vi "Verarbeitung_Unten.vi"(8 "Fehler in":errorcluster, 11 "Cluster in":T2={"Initialisierung"={"Online?"=FALSE, "Grundpfad"=path "", "Kamera Oben"="", "IP-Adresse Flüssiglinse"="", "Flüssiglinse"=refnum, "Kamera Unten"="", "IP-Adresse SPS"="", "SPS-Verbindung"={"TCP Connection Ref"=refnum, "IP address"="", "timeout ms"=5000, "Connected?"=FALSE, "PLC Type"=enum."S7 1200", "Rack S7 400"=0, "Slot S7 400"=0, "PDU Size"=0, "connection semaphore"=refnum}, "IP-Adresse Lichtgitter"="", "Lichtgitter"=refnum, "Skalierungsfaktor"=0.0, "Bilder Oben"=[], "Bild Unten"=refnum, "Bild Ausschnitt Unten"=refnum}, "Einstellungen"={"Gesamtablauf gestartet"=FALSE, "i. O. Bilder speichern"=FALSE, "Bildspeicherung Offline"=FALSE, "Ausgewähltes Offline-Datum"="", "Ausgewähltes Offline-Teil"="", "Speicherpfad Bilder"=path ""}, "Artikeldaten"={"Artikelnummer"="", "Fertigungsauftrag"="", "Muster ISO"=refnum, "Belichtungszeit Referenzmarken"=0.0, "Fokus Referenzmarken"=0.0, "Belichtungszeit ISO"=0.0, "Fokus ISO"=0.0, "Belichtungszeit Unten"=0.0, "Kontaktanzahl"=0, "Aktueller Kontakt"=0, "Kontaktposition"={"x"=0.0, "y"=0.0}, "Winkel ISO"=0.0, "ISO-Muster nicht vorhanden"=FALSE}, "Werte Kamera Oben"={"Koordinatensystem"={"Punkt x-Achse"={"X"=0.0, "Y"=0.0}, "Ursprung"={"X"=0.0, "Y"=0.0}, "Punkt y-Achse"={"X"=0.0, "Y"=0.0}}, "Position Kontakt"={"x"=0.0, "y"=0.0}, "Winkel Kontakt"=0.0}, "Werte Kamera Unten"={"Prüfung Unten n. i. O."=FALSE}, "Werte Lichtgitter"={"Messwerte Referenzmarken"=[], "Mittelpunkt Referenzmarken"={"x"=0.0, "y"=0.0}, "Messwerte Kontakt"=[], "Offset"={"x"=0.0, "y"=0.0}}, "Rückmeldungen"={"Koordinaten ermittelt"=FALSE, "Vermessung Lichtgitter fertig"=FALSE, "Nachkontrolle Kamera Unten fertig"=FALSE}, "Fehler"={"Referenzen nicht gefunden"=FALSE, "Kontakt nicht gefunden"=FALSE, "Referenzen nicht in Lichtgitter"=FALSE, "Kontakt zu groß"=FALSE, "Kontakt zu klein"=FALSE}, "Statistik"={"Statistiken"=[]}, "Timer"={"Timer Start Position"=0, "Timer Start Lichtgitter"=0, "Timer Start Kamera Unten"=0}}) -> (0 "Fehler out":errorcluster, 3 "Cluster out":T2={"Initialisierung"={"Online?"=FALSE, "Grundpfad"=path "", "Kamera Oben"="", "IP-Adresse Flüssiglinse"="", "Flüssiglinse"=refnum, "Kamera Unten"="", "IP-Adresse SPS"="", "SPS-Verbindung"={"TCP Connection Ref"=refnum, "IP address"="", "timeout ms"=5000, "Connected?"=FALSE, "PLC Type"=enum."S7 1200", "Rack S7 400"=0, "Slot S7 400"=0, "PDU Size"=0, "connection semaphore"=refnum}, "IP-Adresse Lichtgitter"="", "Lichtgitter"=refnum, "Skalierungsfaktor"=0.0, "Bilder Oben"=[], "Bild Unten"=refnum, "Bild Ausschnitt Unten"=refnum}, "Einstellungen"={"Gesamtablauf gestartet"=FALSE, "i. O. Bilder speichern"=FALSE, "Bildspeicherung Offline"=FALSE, "Ausgewähltes Offline-Datum"="", "Ausgewähltes Offline-Teil"="", "Speicherpfad Bilder"=path ""}, "Artikeldaten"={"Artikelnummer"="", "Fertigungsauftrag"="", "Muster ISO"=refnum, "Belichtungszeit Referenzmarken"=0.0, "Fokus Referenzmarken"=0.0, "Belichtungszeit ISO"=0.0, "Fokus ISO"=0.0, "Belichtungszeit Unten"=0.0, "Kontaktanzahl"=0, "Aktueller Kontakt"=0, "Kontaktposition"={"x"=0.0, "y"=0.0}, "Winkel ISO"=0.0, "ISO-Muster nicht vorhanden"=FALSE}, "Werte Kamera Oben"={"Koordinatensystem"={"Punkt x-Achse"={"X"=0.0, "Y"=0.0}, "Ursprung"={"X"=0.0, "Y"=0.0}, "Punkt y-Achse"={"X"=0.0, "Y"=0.0}}, "Position Kontakt"={"x"=0.0, "y"=0.0}, "Winkel Kontakt"=0.0}, "Werte Kamera Unten"={"Prüfung Unten n. i. O."=FALSE}, "Werte Lichtgitter"={"Messwerte Referenzmarken"=[], "Mittelpunkt Referenzmarken"={"x"=0.0, "y"=0.0}, "Messwerte Kontakt"=[], "Offset"={"x"=0.0, "y"=0.0}}, "Rückmeldungen"={"Koordinaten ermittelt"=FALSE, "Vermessung Lichtgitter fertig"=FALSE, "Nachkontrolle Kamera Unten fertig"=FALSE}, "Fehler"={"Referenzen nicht gefunden"=FALSE, "Kontakt nicht gefunden"=FALSE, "Referenzen nicht in Lichtgitter"=FALSE, "Kontakt zu groß"=FALSE, "Kontakt zu klein"=FALSE}, "Statistik"={"Statistiken"=[]}, "Timer"={"Timer Start Position"=0, "Timer Start Lichtgitter"=0, "Timer Start Kamera Unten"=0}})   [LabVIEW 2024]
doc: "Prüft ob der Kontakt richtig montiert wurde."
uses:
  Cluster.ctl
  Kontaktmontagemodul.exe/1abvi3w/vi.lib/userDefined/High Color/IMAQdx.ctl
  Kontaktmontagemodul.exe/1abvi3w/vi.lib/DATA AHEAD/SP7/typedefs/S7 Connection.ctl
  Kontaktmontagemodul.exe/1abvi3w/vi.lib/DATA AHEAD/SP7/typedefs/PLC Type.ctl
  Kontaktmontagemodul.exe/1abvi3w/vi.lib/vision/Image Controls.llb/IMAQ Image.ctl
  Koordinatensystem.ctl
  Statistik.ctl
  Kontaktmontagemodul.exe/1abvi3w/vi.lib/vision/Measure.llb/Edge Options.ctl
  Kontaktmontagemodul.exe/1abvi3w/vi.lib/vision/Measure.llb/Edge Polarity.ctl
  Kontaktmontagemodul.exe/1abvi3w/vi.lib/vision/NI_Vision_Development_Module.lvlib
  Kontaktmontagemodul.exe/1abvi3w/vi.lib/DATA AHEAD/SP7/SP7.lvlib
panel:
  out "Image":T1(plugin-control)
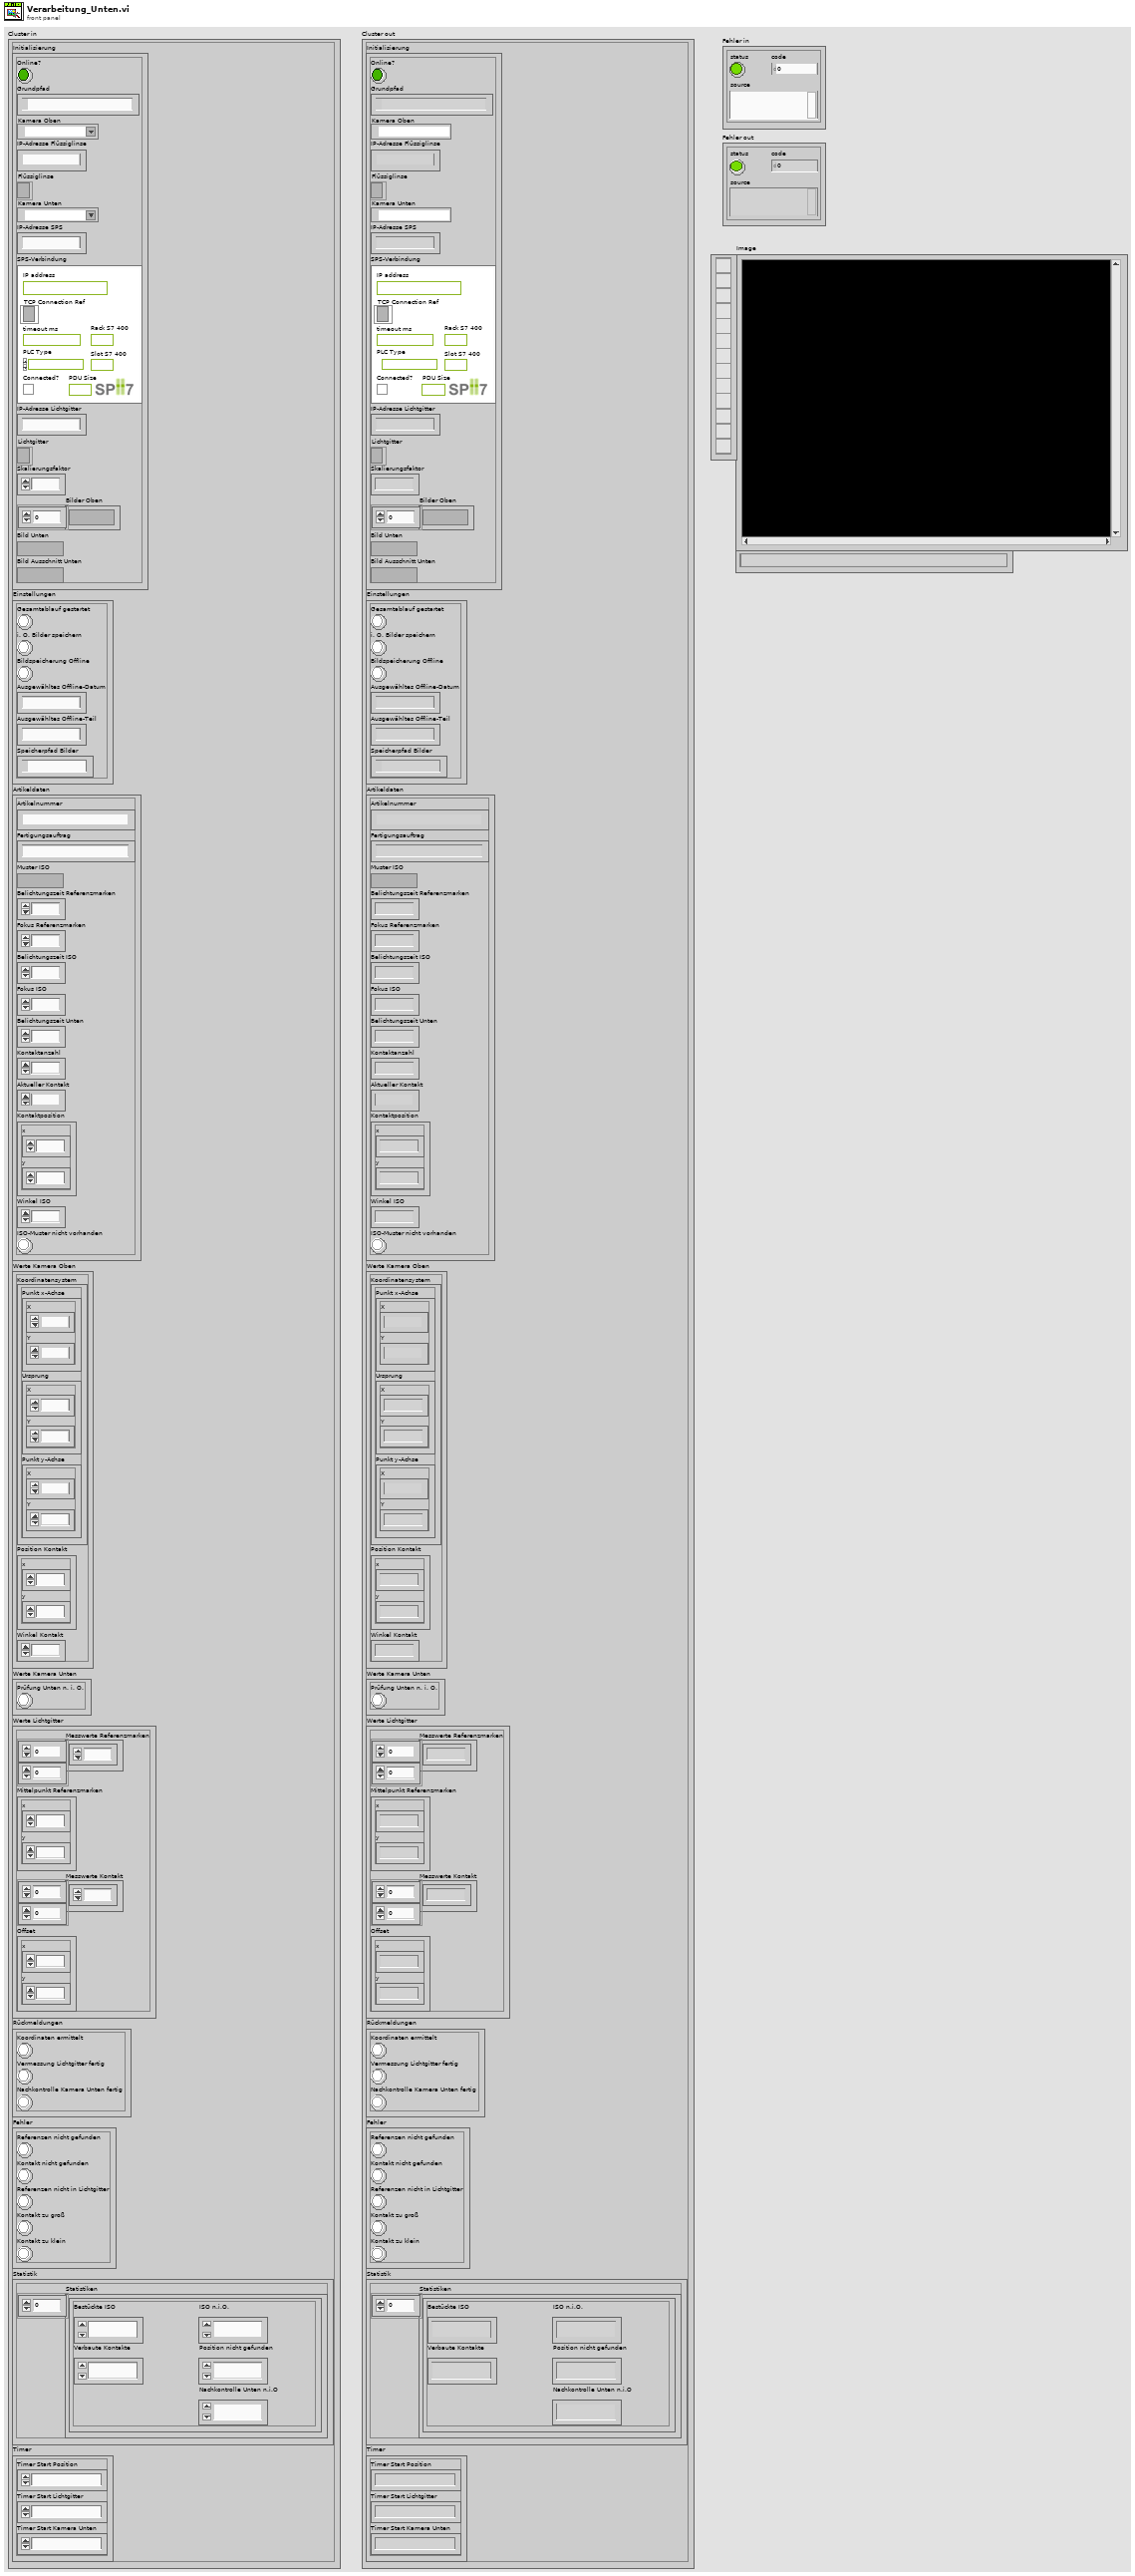
[diagram p1: front panel]
types:
  T1 = typedef "IMAQ Image.ctl" = refnum<image>
  T2 = typedef "Cluster.ctl" = cluster{"Initialisierung":cluster{"Online?":bool, "Grundpfad":path, "Kamera Oben":T3, "IP-Adresse Flüssiglinse":string, "Flüssiglinse":refnum<k5>, "Kamera Unten":T3, "IP-Adresse SPS":string, "SPS-Verbindung":T4, "IP-Adresse Lichtgitter":string, "Lichtgitter":refnum<k5>, "Skalierungsfaktor":dbl, "Bilder Oben":T1[], "Bild Unten":T1, "Bild Ausschnitt Unten":T1}, "Einstellungen":cluster{"Gesamtablauf gestartet":bool, "i. O. Bilder speichern":bool, "Bildspeicherung Offline":bool, "Ausgewähltes Offline-Datum":string, "Ausgewähltes Offline-Teil":string, "Speicherpfad Bilder":path}, "Artikeldaten":cluster{"Artikelnummer":string, "Fertigungsauftrag":string, "Muster ISO":T1, "Belichtungszeit Referenzmarken":dbl, "Fokus Referenzmarken":dbl, "Belichtungszeit ISO":dbl, "Fokus ISO":dbl, "Belichtungszeit Unten":dbl, "Kontaktanzahl":u32, "Aktueller Kontakt":i16, "Kontaktposition":cluster{"x":sgl, "y":sgl}, "Winkel ISO":sgl, "ISO-Muster nicht vorhanden":bool}, "Werte Kamera Oben":cluster{"Koordinatensystem":T7, "Position Kontakt":cluster{"x":dbl, "y":dbl}, "Winkel Kontakt":dbl}, "Werte Kamera Unten":cluster{"Prüfung Unten n. i. O.":bool}, "Werte Lichtgitter":cluster{"Messwerte Referenzmarken":dbl[][], "Mittelpunkt Referenzmarken":cluster{"x":dbl, "y":dbl}, "Messwerte Kontakt":dbl[][], "Offset":cluster{"x":dbl, "y":dbl}}, "Rückmeldungen":cluster{"Koordinaten ermittelt":bool, "Vermessung Lichtgitter fertig":bool, "Nachkontrolle Kamera Unten fertig":bool}, "Fehler":cluster{"Referenzen nicht gefunden":bool, "Kontakt nicht gefunden":bool, "Referenzen nicht in Lichtgitter":bool, "Kontakt zu groß":bool, "Kontakt zu klein":bool}, "Statistik":cluster{"Statistiken":T8[]}, "Timer":cluster{"Timer Start Position":u32, "Timer Start Lichtgitter":u32, "Timer Start Kamera Unten":u32}}
  T3 = typedef "IMAQdx.ctl" = refnum<k21>
  T4 = typedef "SP7.lvlib/S7 Connection.ctl" = cluster{"TCP Connection Ref":refnum<k5>, "IP address":string, "timeout ms":i32, "Connected?":bool, "PLC Type":T5, "Rack S7 400":u8, "Slot S7 400":u8, "PDU Size":u16, "connection semaphore":T6}
  T5 = typedef "SP7.lvlib/PLC Type.ctl" = enum16{"S7 200", "S7 300/400", "S7 1200", "S7 1500", "LOGO!8"}
  T6 = typedef "Semaphore RefNum" = refnum<k1>
  T7 = typedef "Koordinatensystem.ctl" = cluster{"Punkt x-Achse":cluster{"X":sgl, "Y":sgl}, "Ursprung":cluster{"X":sgl, "Y":sgl}, "Punkt y-Achse":cluster{"X":sgl, "Y":sgl}}
  T8 = typedef "Statistik.ctl" = cluster{"Bestückte ISO":u32, "Verbaute Kontakte":u32, "ISO n.i.O.":u32, "Nachkontrolle Unten n.i.O":u32, "Position nicht gefunden":u32}
  T9 = typedef "IMAQ Circle" = cluster{"Center X":i32, "Center Y":i32, "Inner Radius":i32, "Outer Radius":i32, "Start Angle":dbl, "End Angle":dbl}
  T10 = typedef "Edge Options.ctl" = cluster{"Edge Polarity":T11, "Kernel Size":u32, "Width":u32, "Minimum Edge Strength":sgl, "Interpolation Type":enum32{"Zero Order", "Bilinear", "Quadratic", "Cubic", "Bilinear Fixed"}, "Data Processing Method":enum32{"Average", "Median"}}
  T11 = typedef "Edge Polarity.ctl" = u32
  T12 = cluster{"Search  Direction":u32, "Edge Options":T10, "Show Search Area":bool, "Show Search Lines":bool, "Show Edges Found":bool, "Show Result":bool, "Search Area Color":u32, "Search Lines Color":u32, "Edge Locations Color":u32, "Result Color":u32, "Overlay Group Name":string}
  T13 = typedef "ROI Descriptor" = cluster{"Global Rectangle":i32[], "Contours":cluster{"ID":enum32{"External", "Internal"}, "Type":u32, "Coordinates":i32[]}[]}
  T14 = cluster{"Center (Pixels)":cluster{"X":sgl, "Y":sgl}, "Radius (Pixels)":dbl, "Center (Real-World)":cluster{"X":sgl, "Y":sgl}, "Radius (Real-World)":dbl, "Roundness (Real-World)":dbl, "Average Strength":dbl, "Average SNR (dB)":dbl}
  T15 = typedef "IMAQ Rectangle" = cluster{"Left":i32, "Top":i32, "Right":i32, "Bottom":i32, "Rotation":dbl}
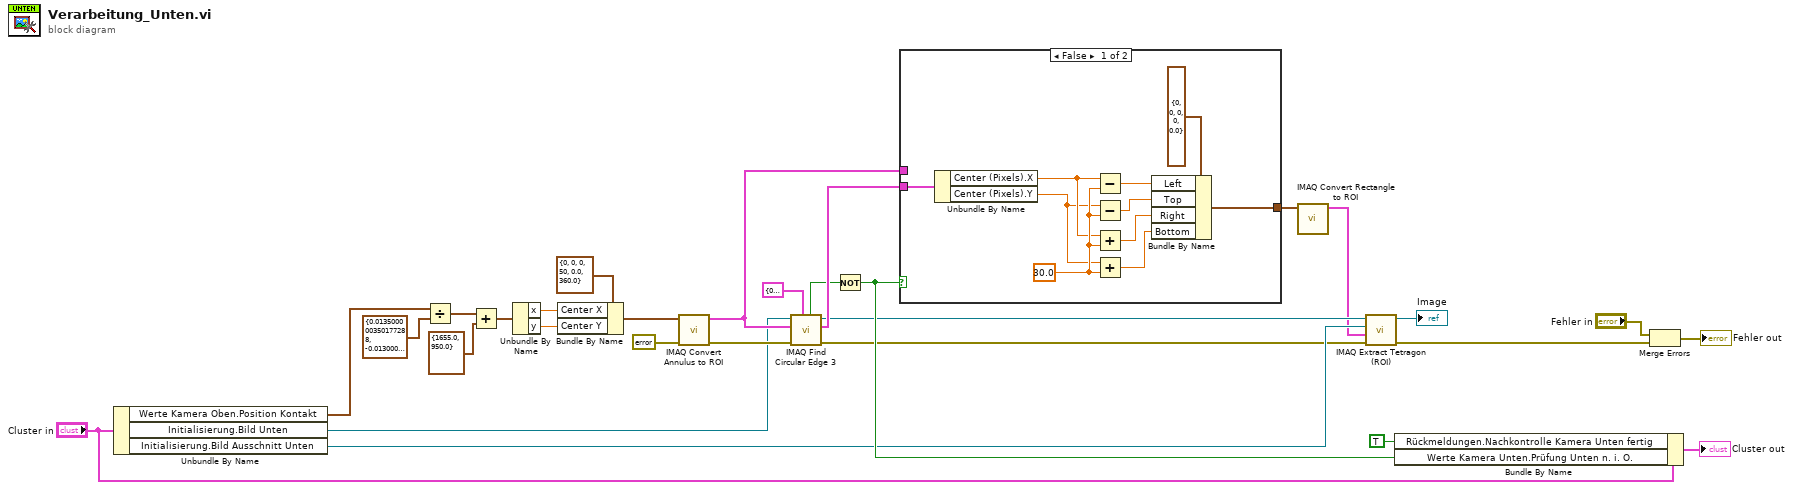
[diagram p0: block diagram]
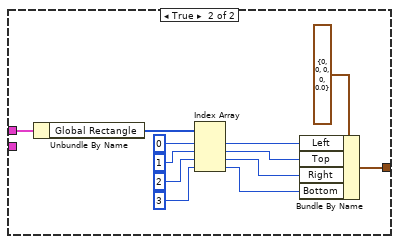
[diagram p2: hidden frame]
diagram:
  n1 = Unbundle By Name("Cluster in") -> ("Werte Kamera Oben.Position Kontakt"=w17:cluster{"x":dbl, "y":dbl}, "Initialisierung.Bild Unten"=w1:T1, "Initialisierung.Bild Ausschnitt Unten"=w9:T1)
  n2 = Divide(x=w17, y=cluster{"x":sgl, "y":sgl} {"x"=0.0135, "y"=-0.013}) -> (x/y=w16:cluster{"x":dbl, "y":dbl})
  n3 = Add(x=w16, y=cluster{"x":dbl, "y":dbl} {"x"=1655.0, "y"=950.0} ("x/y")) -> (x+y=w13:cluster{"x":dbl, "y":dbl})
  n4 = Unbundle By Name(w13) -> ("x"=w12:dbl, "y"=w11:dbl)
  n5 = Bundle By Name(cluster=T9 {"Center X"=0, "Center Y"=0, "Inner Radius"=0, "Outer Radius"=50, "Start Angle"=0.0, "End Angle"=360.0} ("Annulus"), "Center X"=w12, "Center Y"=w11) -> (w10:T9)
  n6 = call "IMAQ Convert Annulus to ROI"("error in (no error)"=errorcluster {"status"=FALSE, "code"=0, "source"=""}, "Annulus"=w10) -> ("error out"=w22:errorcluster, "ROI Descriptor"=w4:T13)  [unwired: 7 in]
  n7 = call "IMAQ Find Circular Edge 3"("Options"=T12 {"Search  Direction"=0, "Edge Options"={"Edge Polarity"=1, "Kernel Size"=3, "Width"=3, "Minimum Edge Strength"=80.0, "Interpolation Type"=enum."Bilinear Fixed", "Data Processing Method"=enum."Average"}, "Show Search Area"=TRUE, "Show Search Lines"=FALSE, "Show Edges Found"=FALSE, "Show Result"=TRUE, "Search Area Color"=65280, "Search Lines Color"=255, "Edge Locations Color"=16776960, "Result Color"=16711680, "Overlay Group Name"=""}, "error in (no error)"=w22, "ROI Descriptor"=w4, "Image"=w1) -> ("error out"=w6:errorcluster, "Fitted Circle"=w23:T14, "Image Out"=w5:T1, "Circle Found"=w19:bool)  [unwired: 3 in, 1 out]
  n8 = Not(x=w19) -> (.not. x?=w18:bool)
  n9 = case shown="False" w18 {
    tunnel: w23 -> [w33 _]
    tunnel: [w30 w50] -> w3
    tunnel: w4 -> [_ w49]
    frame False {
      w34 = sgl 30.0 ("y")
      n10 = Unbundle By Name(w33) -> ("Center (Pixels).X"=w32:sgl, "Center (Pixels).Y"=w31:sgl)
      n11 = Subtract(x=w32, y=w34) -> (x-y=w38:sgl)
      n12 = Subtract(x=w31, y=w34) -> (x-y=w37:sgl)
      n13 = Add(x=w32, y=w34) -> (x+y=w36:sgl)
      n14 = Add(x=w31, y=w34) -> (x+y=w35:sgl)
      n15 = Bundle By Name(cluster=T15 {"Left"=0, "Top"=0, "Right"=0, "Bottom"=0, "Rotation"=0.0} ("Rectangle"), "Left"=w38, "Top"=w37, "Right"=w36, "Bottom"=w35) -> (w30:T15)
    }
    frame True {
      n16 = Unbundle By Name(w49) -> ("Global Rectangle"=w48:i32[])
      n17 = Index Array(array=w48, index #1=0 ("index"), index #2=1 ("index"), index #3=2 ("index"), index #4=3 ("index")) -> (element #1=w43:i32, element #2=w42:i32, element #3=w41:i32, element #4=w40:i32)
      n18 = Bundle By Name(cluster=T15 {"Left"=0, "Top"=0, "Right"=0, "Bottom"=0, "Rotation"=0.0} ("Rectangle"), "Left"=w43, "Top"=w42, "Right"=w41, "Bottom"=w40) -> (w50:T15)
    }
  }
  n19 = call "IMAQ Convert Rectangle to ROI"("Rectangle"=w3) -> ("ROI Descriptor"=w2:T13)  [unwired: 8 in, 1 out]
  n20 = call "IMAQ Extract Tetragon (ROI)"("error in (no error)"=w6, "ROI Descriptor"=w2, "Image Dst"=w9, "Image Src"=w5) -> ("error out"=w7:errorcluster, "Image Dst Out"=→"Image":T1)  [unwired: 6 in]
  n21 = Bundle By Name(cluster="Cluster in", "Rückmeldungen.Nachkontrolle Kamera Unten fertig"=TRUE ("Kamera Unten.Nachkontrolle Kamera Unten fertig"), "Werte Kamera Unten.Prüfung Unten n. i. O."=w18) -> (→"Cluster out":T2)
  n22 = Merge Errors("Fehler in", w7) -> (→"Fehler out":errorcluster)
